vi "GEOM_CorrectCoords.vi"(9 "Amplifiers":T2[](array[typedef]) {"fliped" items=["none", "horizontal", "vertical"]; "type" items=["LL", "LR", "UL", "UR"]}, 10 "readmode":string) -> (1 "correctedReadMode":T1)   [LabVIEW 2016]
uses:
  GEOM_CorrectedFPA.ctl
  GEOM_Amplifier.ctl
  GEOM_AmpType.ctl
  GEOM_ROI.ctl
  GEOM_Coords.ctl
panel:
  in  "Cluster":T1
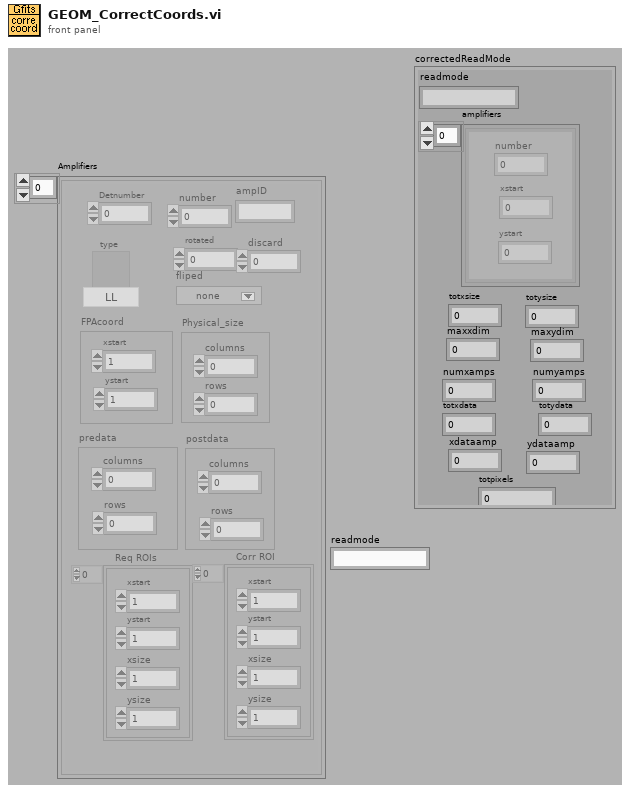
[diagram p1: front panel]
types:
  T1 = typedef "GEOM_CorrectedFPA.ctl" = cluster{"readmode":string, "amplifiers":cluster{"number":i32, "xstart":i32, "ystart":i32}[], "totxsize":i32, "totysize":i32, "maxxdim":i32, "maxydim":i32, "numxamps":i32, "numyamps":i32, "totxdata":i32, "totydata":i32, "xdataamp":i32, "ydataamp":i32, "totpixels":i32}
  T2 = typedef "GEOM_Amplifier.ctl" = cluster{"number":i32, "type":T3, "rotated":i16, "fliped":u16, "FPAcoord":cluster{"xstart":i32, "ystart":i32}, "Physical_size":cluster{"columns":i32, "rows":i32}, "predata":cluster{"columns":i32, "rows":i32}, "postdata":cluster{"columns":i32, "rows":i32}, "Req ROIs":T4, "Corr ROI":T4, "Detnumber":i32, "ampID":string, "discard":i32}
  T3 = typedef "GEOM_AmpType.ctl" = u16
  T4 = typedef "GEOM_ROI.ctl" = T5[]
  T5 = typedef "GEOM_Coords.ctl" = cluster{"xstart":u32, "ystart":u32, "xsize":u32, "ysize":u32}
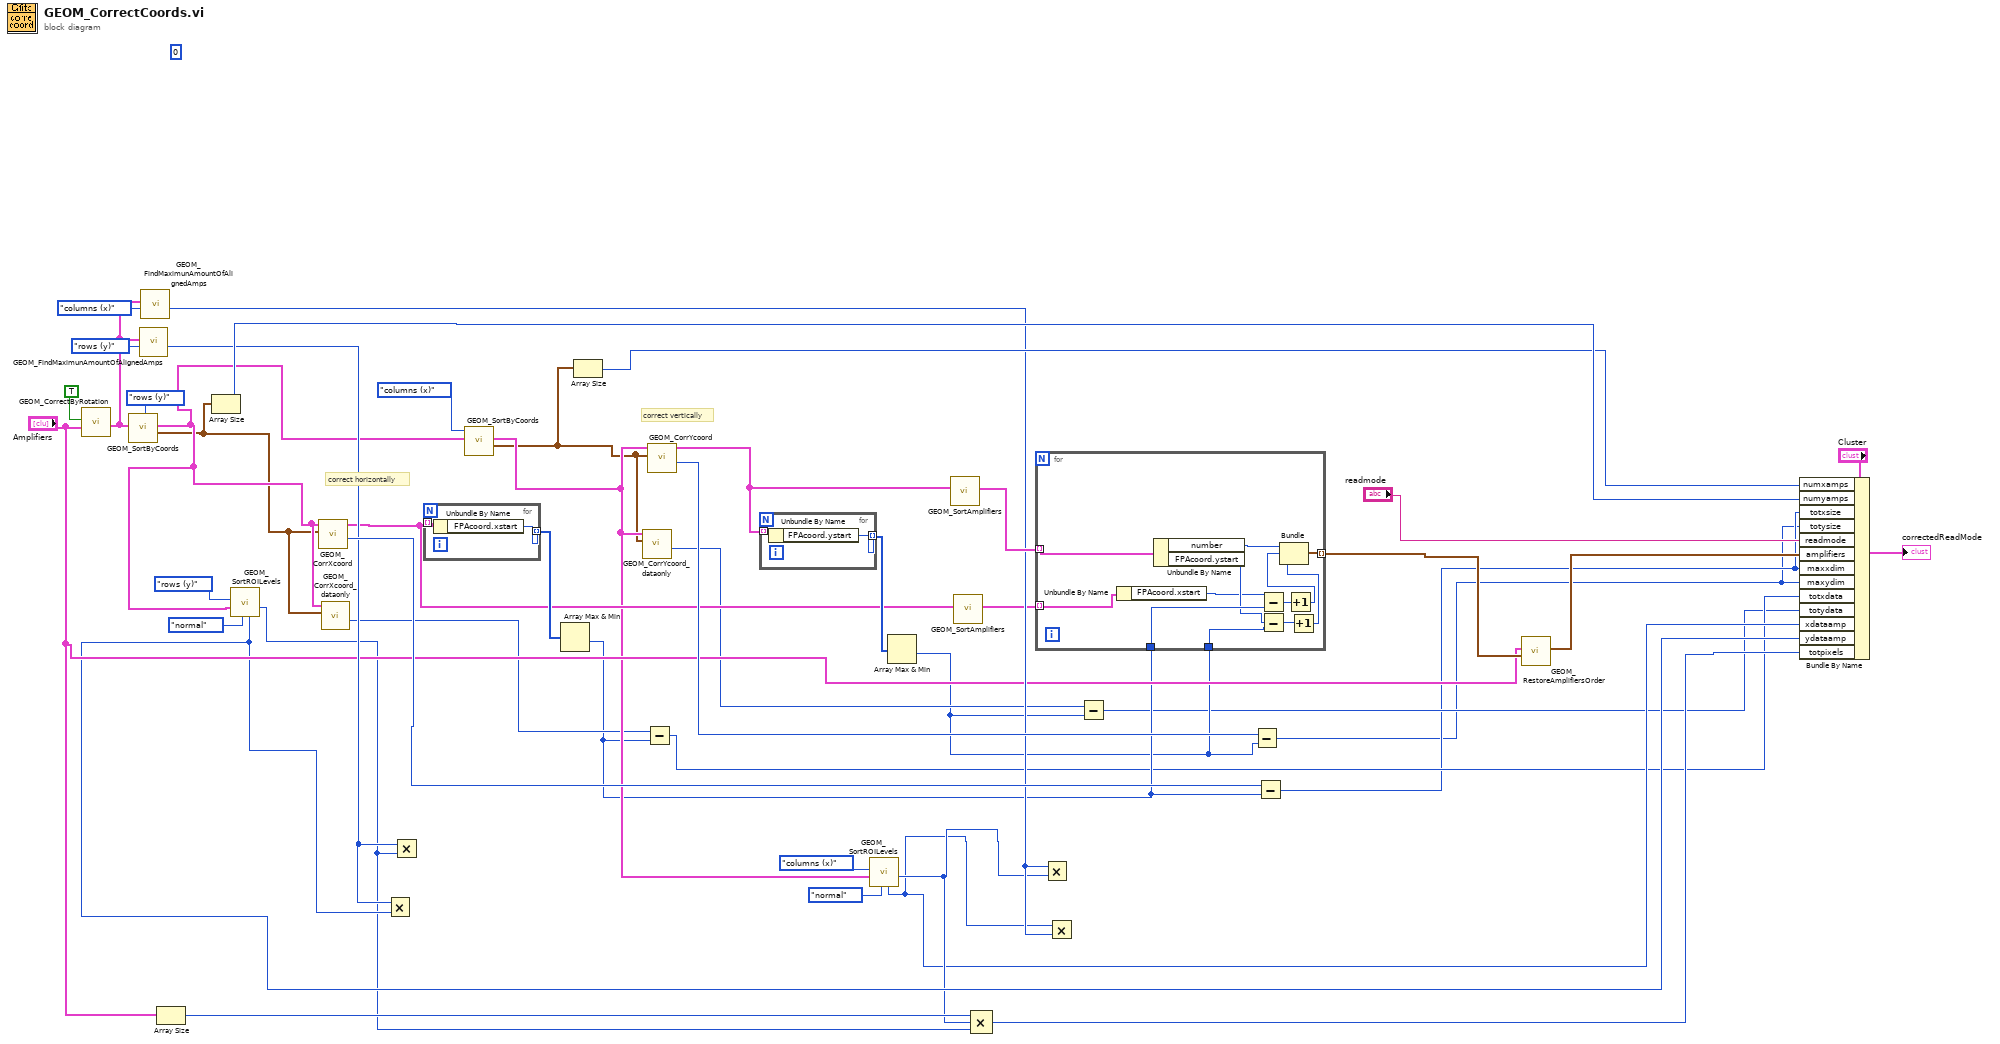
[diagram p0: block diagram]
diagram:
  (unwired) 0
  # "correct vertically"
  # "correct horizontally"
  n1 = call "GEOM_CorrectByRotation.vi"("Amplifiers"="Amplifiers", "rotate ROIs?"=TRUE) -> ("rotated amps"=w27:T2[])  [unwired: 9 out]
  n2 = call "GEOM_SortByCoords.vi"("amplifiers"=w27, "how"=enum16{"rows (y)", "columns (x)"}."rows (y)") -> ("levels"=w11:cluster{"amplifiers":i32, "coord":i32}[], "sorted amplifiers"=w12:T2[])  [unwired: 8 out]
  n3 = call "GEOM_FindMaximunAmountOfAlignedAmps.vi"("how"=enum16{"rows (y)", "columns (x)"}."rows (y)", "amplifiers"=w27) -> ("maxalignedamps"=w24:i32)  [unwired: 9 out]
  n4 = call "GEOM_FindMaximunAmountOfAlignedAmps.vi"("how"=enum16{"rows (y)", "columns (x)"}."columns (x)", "amplifiers"=w27) -> ("maxalignedamps"=w25:i32)  [unwired: 9 out]
  n5 = Array Size(array="Amplifiers") -> (size(s)=w34:i32)
  n6 = Array Size(array=w11) -> (size(s)=w39:i32)
  n7 = call "GEOM_SortROILevels.vi"("type"=enum16{"any", "normal", "rotated"}."normal", "amplifiers"=w12, "how"=enum16{"rows (y)", "columns (x)"}."rows (y)") -> ("totpix"=w16:u32, "totdata"=w17:i32)  [unwired: 1 in, 6 out]
  n8 = call "GEOM_CorrXcoord.vi"("levels"=w11, "Array"=w12) -> ("xcoord"=w32:u32, "Array 2"=w20:T2[])  [unwired: 8 out]
  n9 = call "GEOM_CorrXcoord_dataonly.vi"("levels"=w11, "Array"=w12) -> ("xcoord"=w8:u32)  [unwired: 9 out]
  n10 = Multiply(x=w24, y=w17) -> ()  [unwired: 1 out]
  n11 = Multiply(x=w24, y=w16) -> ()  [unwired: 1 out]
  n12 = for {
    tunnel: w20 -> [w48] mode=indexing
    tunnel: [w47] -> w36 mode=indexing
    n13 = Unbundle By Name(w48) -> ("FPAcoord.xstart"=w47:i32)
  }
  n14 = call "GEOM_SortByCoords.vi"("amplifiers"=w12, "how"=enum16{"rows (y)", "columns (x)"}."columns (x)") -> ("levels"=w9:cluster{"amplifiers":i32, "coord":i32}[], "sorted amplifiers"=w10:T2[])  [unwired: 8 out]
  n15 = Array Max & Min(array=w36) -> (min value=w7:i32)  [unwired: 3 out]
  n16 = Array Size(array=w9) -> (size(s)=w29:i32)
  n17 = call "GEOM_CorrYcoord_dataonly.vi"("levels"=w9, "Array"=w10) -> ("ycoord"=w5:u32)  [unwired: 9 out]
  n18 = Subtract(x=w8, y=w7) -> (x-y=w6:u32)
  n19 = call "GEOM_CorrYcoord.vi"("levels"=w9, "Array"=w10) -> ("ycoord"=w30:u32, "Array 2"=w31:T2[])  [unwired: 8 out]
  n20 = for {
    tunnel: w31 -> [w50] mode=indexing
    tunnel: [w49] -> w35 mode=indexing
    n21 = Unbundle By Name(w50) -> ("FPAcoord.ystart"=w49:i32)
  }
  n22 = call "GEOM_SortROILevels.vi"("type"=enum16{"any", "normal", "rotated"}."normal", "amplifiers"=w10, "how"=enum16{"rows (y)", "columns (x)"}."columns (x)") -> ("totpix"=w14:u32, "totdata"=w13:i32)  [unwired: 1 in, 6 out]
  n23 = Array Max & Min(array=w35) -> (min value=w4:i32)  [unwired: 3 out]
  n24 = call "GEOM_SortAmplifiers.vi"("amplifiers"=w31) -> ("sorted amplifiers"=w44:T2[])  [unwired: 10 out]
  n25 = call "GEOM_SortAmplifiers.vi"("amplifiers"=w20) -> ("sorted amplifiers"=w19:T2[])  [unwired: 10 out]
  n26 = Compound Arithmetic op=MULTIPLY(w34, w14, w16) -> (w33:u32)
  n27 = for {
    tunnel: w44 -> [w62] mode=indexing
    tunnel: [w60] -> w23 mode=indexing
    tunnel: w4 -> [w55]
    tunnel: w7 -> [w59]
    tunnel: w19 -> [w52] mode=indexing
    n28 = Unbundle By Name(w52) -> ("FPAcoord.xstart"=w51:i32)
    n29 = Unbundle By Name(w62) -> ("number"=w61:i32, "FPAcoord.ystart"=w56:i32)
    n30 = Subtract(x=w51, y=w59) -> (x-y=w58:i32)
    n31 = Subtract(x=w56, y=w55) -> (x-y=w54:i32)
    n32 = Increment(x=w58) -> (x+1=w57:i32)
    n33 = Increment(x=w54) -> (x+1=w53:i32)
    n34 = Bundle("number"=w61, w57, w53) -> (w60:cluster{"number":i32, i32, i32})  [unwired: 1 out]
  }
  n35 = Multiply(x=w25, y=w14) -> ()  [unwired: 1 out]
  n36 = Multiply(x=w13, y=w25) -> ()  [unwired: 1 out]
  n37 = Subtract(x=w5, y=w4) -> (x-y=w3:u32)
  n38 = Subtract(x=w30, y=w4) -> (x-y=w1:u32)
  n39 = Subtract(x=w32, y=w7) -> (x-y=w2:u32)
  n40 = call "GEOM_RestoreAmplifiersOrder.vi"("sorted amps"=w23, "orig amplifiers"="Amplifiers") -> ("restored order"=w21:cluster{"number":i32, i32, i32}[])  [unwired: 9 out]
  n41 = Bundle By Name(cluster="Cluster", "numxamps"=w29, "numyamps"=w39, "totxsize"=w2, "totysize"=w1, "readmode"="readmode", "amplifiers"=w21, "maxxdim"=w2, "maxydim"=w1, "totxdata"=w6, "totydata"=w3, "xdataamp"=w13, "ydataamp"=w17, "totpixels"=w33) -> (→"correctedReadMode":T1)
